vi "Initialize.vi"(6 "Current Units":string, 8 "error in (no error)":errorcluster, 9 "Encoder Resolution":string, 10 "Axis Letter":string, 11 "Axis in":refnum<class "Axis.lvclass">) -> (0 "error out":errorcluster, 3 "Axis out":refnum<class "Axis.lvclass">)   [LabVIEW 2019, in "Axis.lvclass"]
uses:
  Axis.lvclass
  Axis.lvclass/Axis.ctl
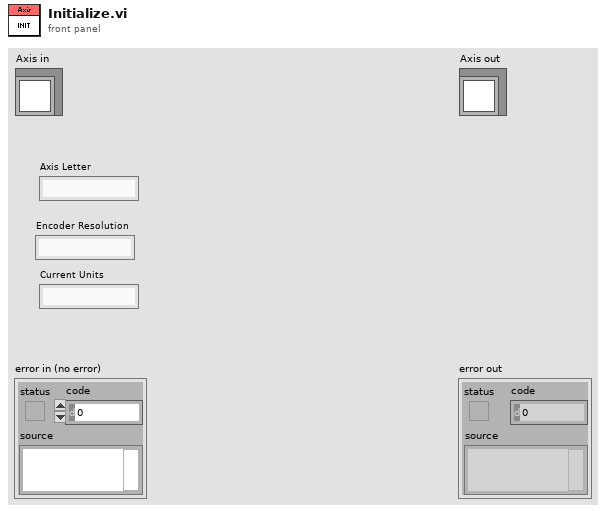
[diagram p1: front panel]
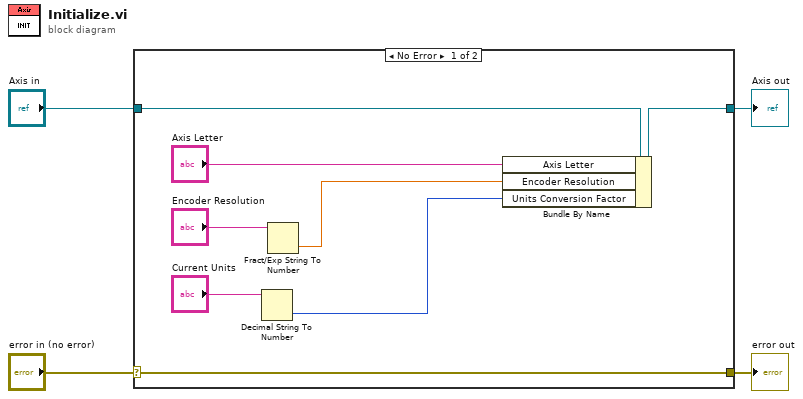
[diagram p0: block diagram]
diagram:
  n1 = case shown="No Error" "error in (no error)" {
    selector: "error in (no error)" -> [w12 w14]
    tunnel: [w12 w14] -> w3
    tunnel: [w6 w13] -> w1
    tunnel: "Axis in" -> [w11 w13]
    frame No Error {
      n2 = Decimal String To Number(string="Current Units") -> (number=w5:i32)  [unwired: 2 in, 1 out]
      n3 = Fract/Exp String To Number(string="Encoder Resolution") -> (number=w7:dbl)  [unwired: 3 in, 1 out]
      n4 = Bundle By Name(cluster=w11, "Axis Letter"="Axis Letter", "Encoder Resolution"=w7, "Units Conversion Factor"=w5) -> (w6:refnum<class "Axis.lvclass">)
    }
    frame Error {
    }
  }
  "error out" <- w3
  "Axis out" <- w1
